vi "Write Path Switch.lvclass.vi"(10 "Path Switch.lvclass":refnum<class "Path Switch.lvclass">, 11 "PathControl in":refnum<class "PathControl.lvclass">) -> (3 "PathControl out":refnum<class "PathControl.lvclass">)   [LabVIEW 2020, in "PathControl.lvclass"]
uses:
  PathControl.lvclass
  Instruments/Path Switch/Path Switch.lvclass
  PathControl.lvclass/PathControl.ctl
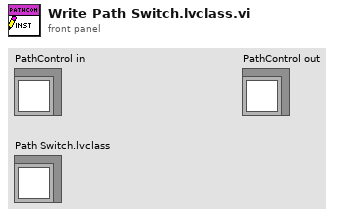
[diagram p1: front panel]
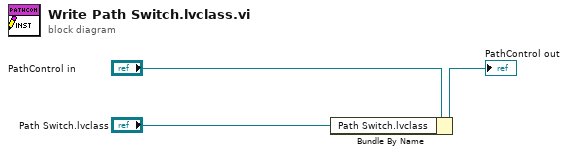
[diagram p0: block diagram]
diagram:
  n1 = Bundle By Name(cluster="PathControl in", "Path Switch.lvclass"="Path Switch.lvclass") -> (→"PathControl out":refnum<class "PathControl.lvclass">)
